vi "MainPanel.vi"() -> ()   [LabVIEW 2024]
panel:
  in  "Diagnose_Panel":enum32{"MAIN_PANEL", "COM_HANDLER"}(tab)
  in  "error name (type empty to clear)":string
  in  "Remove error":bool
  out "cem_off":bool
  out "cem_on":bool
  in  "UPDATE":bool
  in  "IGN_EN\nOn/Off":bool
  out "1_IGN":bool
  out "0_OFF":bool
  in  "GEAR SFT":i8(slide) scale=-1.0..6.0
  in  "PEDAL":i8(slide) scale=0.0..100.0
  out "power/torque/speed- graph":cluster{"power":i32, "torque":i32, "speed":u64}(graph)
  out "off":bool=TRUE
  out "on":bool
  in  "Send key check resp (auth req on(br.red)/off)":bool
  out "Security access status":string="N/A"
  out "?":string="    OCTAVIA III DIAGNOSE SERVICE"
  in  "STOP DIAG_SERVICE":bool
  in  "milliseconds to wait":u32=200
  out "key":u64
  out "seed":u64
  in  "GET security acces data":bool
  in  "Cluster":T1
  out "stop":bool=TRUE
  out "run":bool
  out "engine_info.speed":u64(knob) caption="km/h" scale=0.0..260.0 scale format="%#_3g"
  out "engine_info.rpm":u64(knob) caption="rpm" scale=0.0..6000.0 scale format="%#_5g"
  out "engine_info.coolant_temp":i32(slide) caption="°C" scale=50.0..130.0
  in  "Start/Stop measurement":bool
  out "engine_info.fuel_consumtion":dbl(slide) caption="l/100km" scale=0.0..30.0
  out "power_supply":dbl(knob) caption="V" scale=0.0..18.0
  out "ign_stat":string
  out "torque (Nm)":i32
  out "power (hp)":i32
  out "rpm":u64
  out "speed (km/h)":u64
  out "pedal_lvl (%)":i32
  out "GEAR":string
  out "fuel_consumtion (l/100km)":dbl
  out "oil_level (%)":i32
  out "coolant_level (%)":i32
  out "coolant_temp (°C)":i32
  out "voltage (V)":dbl
  in  "Set_Ped_EN":bool
  in  "Chng_Gear_EN":bool
  in  "IGNITION\nOFF_0/IGN_1":bool
  out "error_memory":string
  out "error_log":string
  out "error_input":string
  in  "update_err_mem":bool
  in  "update_err_input":bool
  in  "update_err_log":bool
  in  "CLR ERR MEM":bool
  in  "CLR ERR LOG":bool
  in  "CLR ERR INPUT":bool
  out "ceg_on":bool
  out "ceg_off":bool
  out "cei_on":bool
  out "cei_off":bool
  in  "oil_level":i32
  in  "cool_lvl":i32
  in  "voltage":i32
  in  "set cool lvl":bool
  in  "set voltage":bool
  in  "set oil lvl":bool
  in  "Array":cluster{"String":string, "Boolean":bool}[](array[cluster])=[{"String"="EngErr_RpmSensorMalfunction", "Boolean"=FALSE}, {"String"="EngErr_FuelConsmUnav", "Boolean"=FALSE}, {"String"="EngErr_SpdmtrFault\n                0xE0112:  \"EngErr_SpdmtrFault\",\n", "Boolean"=FALSE}, {"String"="EngErr_EngCoolOverheat", "Boolean"=FALSE}, {"String"="EngErr_OilLvlLow", "Boolean"=FALSE}, {"String"="EngErr_CoolLvlLow", "Boolean"=FALSE}, {"String"="EngErr_IgnMalfunction", "Boolean"=FALSE}, {"String"="EngErr_Malfunction_Injector_1", "Boolean"=FALSE}, {"String"="EngErr_Malfunction_Injector_2", "Boolean"=FALSE}, {"String"="EngErr_Malfunction_Injector_3", "Boolean"=FALSE}, {"String"="EngErr_Malfunction_Injector_4", "Boolean"=FALSE}, {"String"="ComErr_CanErr_LossOfComm", "Boolean"=FALSE}, {"String"="ComErr_CanErr_Overvoltage", "Boolean"=FALSE}, {"String"="ComErr_CanErr_Undervoltage", "Boolean"=FALSE}, {"String"="ElErr_Overvoltage", "Boolean"=FALSE}, {"String"="ElErr_Undervoltage", "Boolean"=FALSE}]
  in  "Inject errors":bool
  out "Injected":bool
  out "no.of.errs":i32
  out "update_error_memory":bool
  out "update_error_log":bool
  out "update_error_input":bool
  out "put_ign_stat_header":string="N/A"
  out "get_ignition_status_header":string
  out "get_sec_stat_header":string="N/A"
  in  "API_KEY":string="cheia04042025tema2restfulapi"
  out "get_key_headers":string="N/A"
  out "put_send_key_header":string="N/A"
  out "get_engine_info_header":string
  out "get_power_supply_header":string
  out "put_gear_change_header":string="N/A"
  out "put_pedal_lvl_header":string="N/A"
  out "get_error_memory_header":string
  out "get_error_log_header":string
  out "get_error_input_header":string
  out "delete_error_memory_header":string="N/A"
  out "delete_error_log_header":string="N/A"
  out "delete_error_inj_header":string="N/A"
  out "put_manipulate_oil_lvl_header":string="N/A"
  out "put_manipulate_voltage_header":string="N/A"
  out "put_manipulate_coolant_lvl_header":string="N/A"
  out "post_error_input_header":string="N/A"
  out "delete_clear_specific_error_header":string="N/A"
  # "Error manager"
  # "COCKPIT"
  # "-UPDATE/DELETE-"
  # "enabled/disabled"
  # "Security access"
  # "-UPDATE/DELETE-"
  # "enabled/disabled"
  # "-UPDATE/DELETE-"
  # "enabled/disabled"
  # "Delete specific error"
  # "CONTROLS (PUT)"
  # "Params"
  # "Manipulate values"
  # "to set errors"
  # "oil: 0-150 %\ncool: 0-150 %\nvoltage: 0-20 V"
  # "Error Injection(POST)"
  # "Click red circle\nto enable/disable\nauthentification\nrequest."
  # "GET REQUESTS"
  # "PUT REQUESTS"
  # "DELETE REQUESTS"
  # "DELETE REQUESTS"
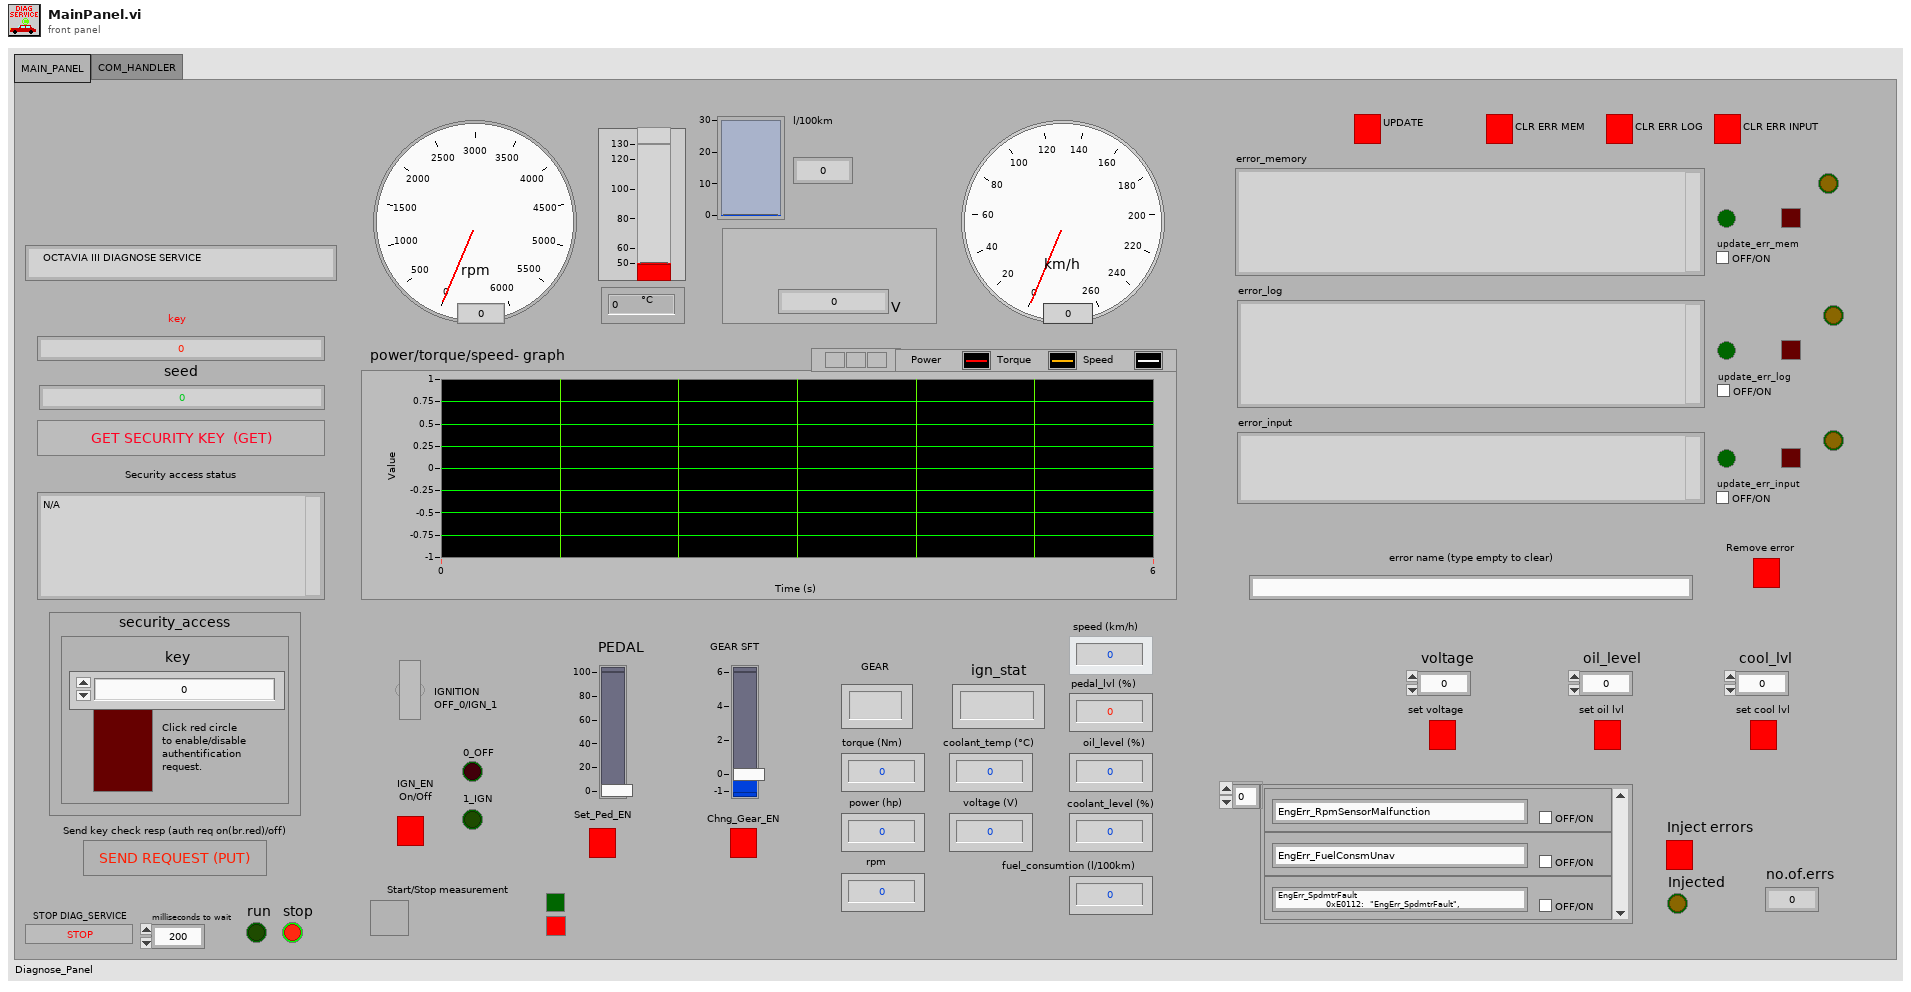
[diagram p1: front panel]
types:
  T1 = cluster{"security_access":cluster{"auth_request":bool, "key":u64}}
  T2 = cluster{"engine_info":cluster{"rpm":u64, "speed":u64, "gear":string, "power":i32, "torque":i32, "fuel_consumtion":dbl, "coolant_temp":i32, "coolant_level":i32, "oil_level":i32, "pedal_lvl":i32}}
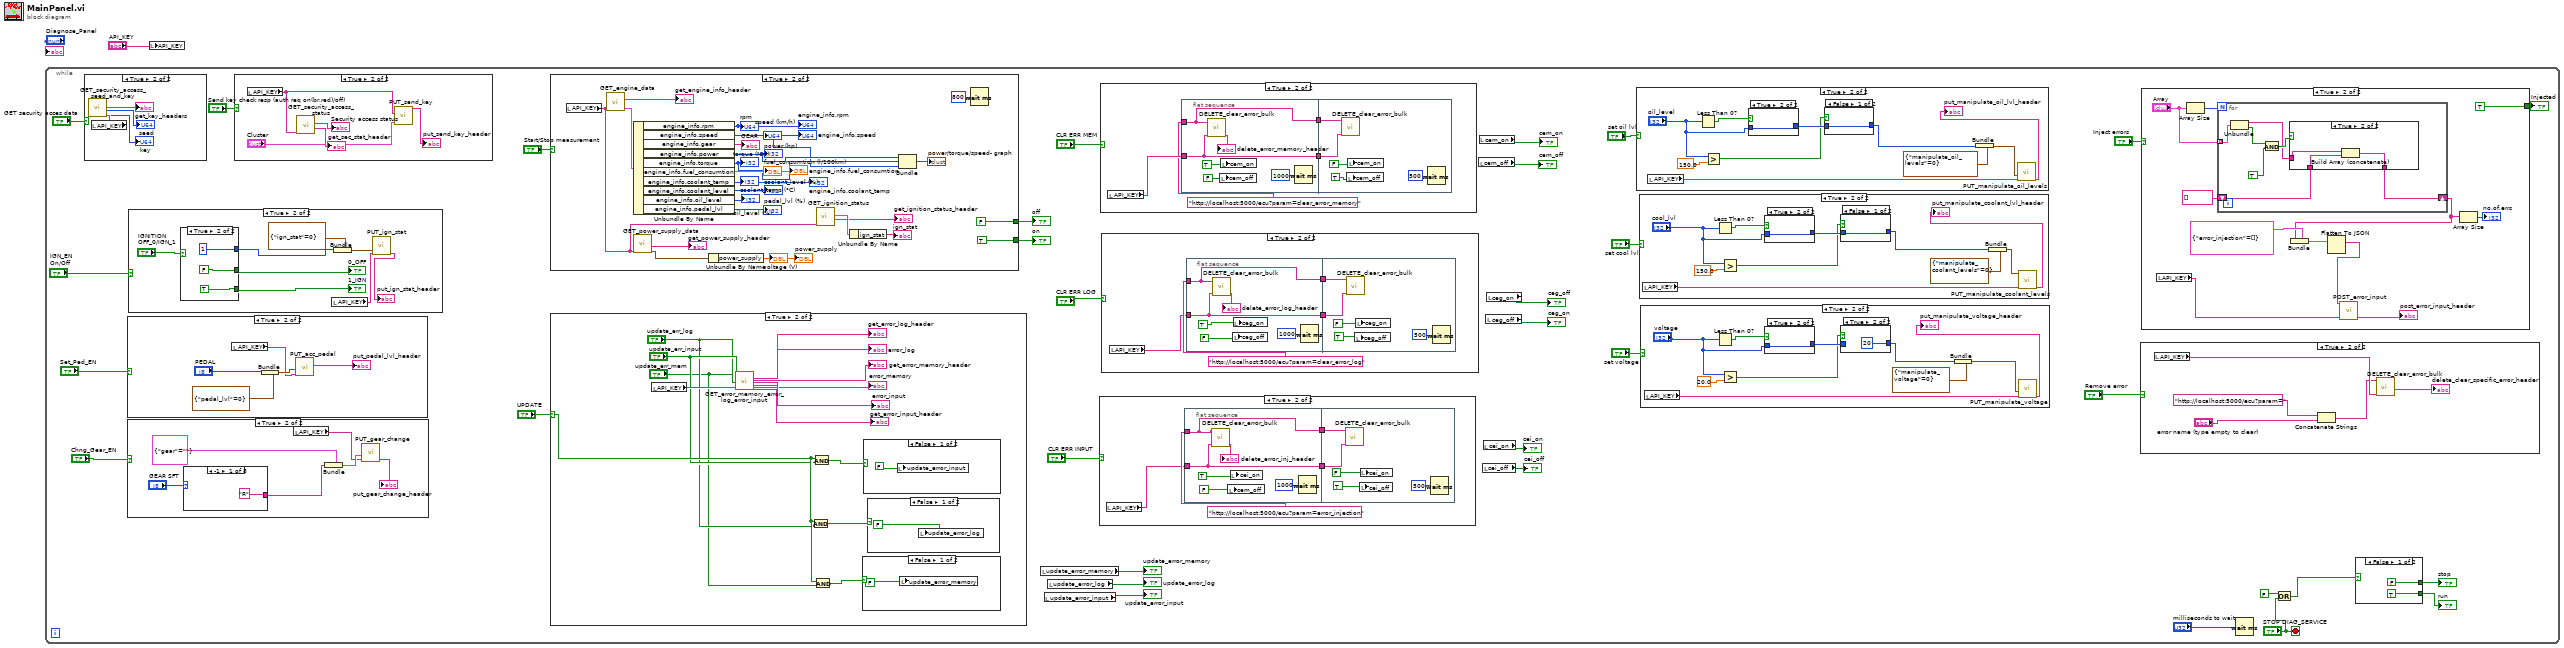
[diagram p0: block diagram]
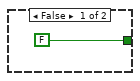
[diagram p3: hidden frame]
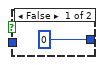
[diagram p7: hidden frame]
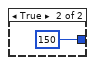
[diagram p9: hidden frame]
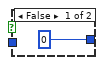
[diagram p10: hidden frame]
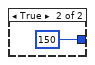
[diagram p12: hidden frame]
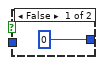
[diagram p13: hidden frame]
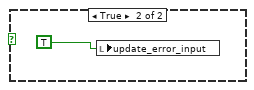
[diagram p18: hidden frame]
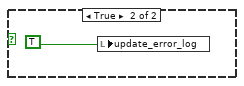
[diagram p19: hidden frame]
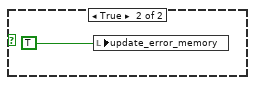
[diagram p20: hidden frame]
diagram:
  n1 = while {
    stop <- "STOP DIAG_SERVICE" stop-if-true
    n2 = case shown="True" "GET security acces data" {
      frame False {
      }
      frame True {
        n3 = local read "API_KEY"() -> (w240:string)
        n4 = call "GET_security_access_seed_and_key.vi"("API Key"=w240) -> ("key"=→"key":u64, "seed"=→"seed":u64, "headers"=→"get_key_headers":string)  [unwired: 5 in, 3 out]
      }
    }
    n5 = case shown="True" "Set_Ped_EN" {
      frame False {
      }
      frame True {
        n6 = local read "API_KEY"() -> (w184:string)
        n7 = Bundle(cluster=cluster{"pedal_lvl":i8} {"pedal_lvl"=0}, "pedal_lvl"="PEDAL") -> (w187:cluster{"pedal_lvl":i8})
        n8 = call "PUT_acc_pedal.vi"("API Key"=w184, "Cluster"=w187) -> ("headers"=→"put_pedal_lvl_header":string)  [unwired: 7 in, 2 out]
      }
    }
    n9 = case shown="True" "Chng_Gear_EN" {
      frame False {
      }
      frame True {
        n10 = case shown="-1" "GEAR SFT" {
          tunnel: ["R" "N" "1" "2" "3" "4" "5" "6"] -> w174
          frame -1 {
          }
          frame 0, Default {
          }
          frame 1 {
          }
          frame 2 {
          }
          frame 3 {
          }
          frame 4 {
          }
          frame 5 {
          }
          frame 6 {
          }
        }
        n11 = local read "API_KEY"() -> (w170:string)
        n12 = Bundle(cluster=cluster{"gear":string} {"gear"=""}, "gear"=w174) -> (w173:cluster{"gear":string})
        n13 = call "PUT_gear_change.vi"("API Key"=w170, "Cluster"=w173) -> ("headers"=→"put_gear_change_header":string)  [unwired: 7 in, 2 out]
      }
    }
    n14 = case shown="True" "IGN_EN\nOn/Off" {
      frame False {
      }
      frame True {
        n15 = case shown="True" "IGNITION\nOFF_0/IGN_1" {
          tunnel: [0 1] -> w192
          tunnel: [TRUE FALSE] -> w191
          tunnel: [FALSE TRUE] -> w195
          frame False {
          }
          frame True {
          }
        }
        "0_OFF" <- w191
        "1_IGN" <- w195
        n16 = local read "API_KEY"() -> (w190:string)
        n17 = Bundle(cluster=cluster{"ign_stat":i32} {"ign_stat"=0}, "ign_stat"=w192) -> (w193:cluster{"ign_stat":i32})
        n18 = call "PUT_ign_stat.vi"("API Key"=w190, "Cluster"=w193) -> ("headers"=→"put_ign_stat_header":string)  [unwired: 7 in, 2 out]
      }
    }
    n19 = case shown="True" "Send key check resp (auth req on(br.red)/off)" {
      frame False {
      }
      frame True {
        n20 = local read "API_KEY"() -> (w232:string)
        n21 = call "GET_security_access_status.vi"("API Key"=w232) -> ("headers"=→"get_sec_stat_header":string, "body"=→"Security access status":string)  [unwired: 8 in, 1 out]
        n22 = call "PUT_send_key.vi"("Cluster"="Cluster", "API Key"=w232) -> ("headers"=→"put_send_key_header":string)  [unwired: 8 in, 1 out]
      }
    }
    n23 = case shown="True" "Start/Stop measurement" {
      tunnel: [TRUE FALSE] -> w25
      tunnel: [FALSE TRUE] -> w24
      frame False {
      }
      frame True {
        n24 = local read "API_KEY"() -> (w209:string)
        n25 = call "GET_engine_data.vi"("API Key"=w209) -> ("engine info"=w226:T2, "headers"=→"get_engine_info_header":string)  [unwired: 8 in, 1 out]
        n26 = call "GET_power_supply_data.vi"("API Key"=w209) -> ("power_suppy"=w216:cluster{"power_supply":dbl}, "headers"=→"get_power_supply_header":string)  [unwired: 8 in, 1 out]
        n27 = Unbundle By Name(w226) -> ("engine_info.rpm"=→"rpm" →"engine_info.rpm":u64, "engine_info.speed"=w212:u64, "engine_info.gear"=→"GEAR":string, "engine_info.power"=w214:i32, "engine_info.torque"=w213:i32, "engine_info.fuel_consumtion"=→"fuel_consumtion (l/100km)" →"engine_info.fuel_consumtion":dbl, "engine_info.coolant_temp"=→"coolant_temp (°C)" →"engine_info.coolant_temp":i32, "engine_info.coolant_level"=→"coolant_level (%)":i32, "engine_info.oil_level"=→"oil_level (%)":i32, "engine_info.pedal_lvl"=→"pedal_lvl (%)":i32)
        "speed (km/h)" <- w212
        "power (hp)" <- w214
        "torque (Nm)" <- w213
        "engine_info.speed" <- w212
        n28 = Unbundle By Name(w216) -> ("power_supply"=→"voltage (V)" →"power_supply":dbl)
        n29 = call "GET_ignition_status.vi"("API Key"=w209) -> ("headers"=→"get_ignition_status_header":string, "ign_stat"=w208:cluster{"ign_stat":string})  [unwired: 8 in, 1 out]
        n30 = Unbundle By Name(w208) -> ("ign_stat"=→"ign_stat":string)
        n31 = Bundle("power"=w214, "torque"=w213, "speed"=w212) -> (→"power/torque/speed- graph":cluster{"power":i32, "torque":i32, "speed":u64})  [unwired: 1 in]
        n32 = Wait (ms)(milliseconds to wait=u32 800) -> ()  [unwired: 1 out]
      }
    }
    "on" <- w24
    "off" <- w25
    n33 = case shown="True" "UPDATE" {
      selector: "UPDATE" -> [_ w156]
      frame False {
      }
      frame True {
        n34 = local read "API_KEY"() -> (w157:string)
        n35 = call "GET_error_memory_error_log_error_input.vi"("update_err_log"="update_err_log", "update_err_input"="update_err_input", "update_err_mem"="update_err_mem", "API Key"=w157) -> ("body_error_log"=→"error_log":string, "get_error_memory"=→"get_error_memory_header":string, "body_error_input"=→"error_input":string, "get_error_log_header"=→"get_error_log_header":string, "body_error_memory"=→"error_memory":string, "get_error_input_header"=→"get_error_input_header":string)  [unwired: 18 in]
        n36 = And(x=w156, y="update_err_log") -> (x .and. y?=w154:bool)
        n37 = And(x=w156, y="update_err_input") -> (x .and. y?=w155:bool)
        n38 = And(x=w156, y="update_err_mem") -> (x .and. y?=w153:bool)
        n39 = case shown="False" w153 {
          frame False {
            n40 = local write "update_error_memory"(FALSE) -> ()
          }
          frame True {
            n41 = local write "update_error_memory"(TRUE) -> ()
          }
        }
        n42 = case shown="False" w155 {
          frame False {
            n43 = local write "update_error_input"(FALSE) -> ()
          }
          frame True {
            n44 = local write "update_error_input"(TRUE) -> ()
          }
        }
        n45 = case shown="False" w154 {
          frame False {
            n46 = local write "update_error_log"(FALSE) -> ()
          }
          frame True {
            n47 = local write "update_error_log"(TRUE) -> ()
          }
        }
      }
    }
    n48 = local read "update_error_memory"() -> (→"update_error_memory":bool)
    n49 = local read "update_error_input"() -> (→"update_error_input":bool)
    n50 = local read "update_error_log"() -> (→"update_error_log":bool)
    n51 = case shown="True" "CLR ERR INPUT" {
      frame False {
      }
      frame True {
        n52 = local read "API_KEY"() -> (w105:string)
        n53 = flat-sequence {
          tunnel: w105 -> [w114]
          tunnel: [w114] -> w108
          tunnel: "http://localhost:5000/ecu?param=error_injection" ("url") -> [w111]
          tunnel: [w111] -> w107
          tunnel: w108 -> [w119]
          tunnel: w107 -> [w117]
          frame #0 {
            n54 = call "DELETE_clear_error_bulk.vi"("API Key"=w114, "url"=w111) -> ("delete_error_"=→"delete_error_inj_header":string)  [unwired: 8 in, 1 out]
            n55 = local write "cem_off"(FALSE) -> ()
            n56 = local write "cei_on"(TRUE) -> ()
            n57 = Wait (ms)(milliseconds to wait=u32 1000) -> ()  [unwired: 1 out]
          }
          frame #1 {
            n58 = call "DELETE_clear_error_bulk.vi"("API Key"=w119, "url"=w117) -> ()  [unwired: 8 in, 2 out]
            n59 = local write "cei_off"(TRUE) -> ()
            n60 = local write "cei_on"(FALSE) -> ()
            n61 = Wait (ms)(milliseconds to wait=u32 500) -> ()  [unwired: 1 out]
          }
        }
      }
    }
    n62 = case shown="True" "CLR ERR MEM" {
      frame False {
      }
      frame True {
        n63 = local read "API_KEY"() -> (w138:string)
        n64 = flat-sequence {
          tunnel: w138 -> [w144]
          tunnel: [w144] -> w137
          tunnel: "http://localhost:5000/ecu?param=clear_error_memory" ("url") -> [w141]
          tunnel: [w141] -> w135
          tunnel: w137 -> [w149]
          tunnel: w135 -> [w147]
          frame #0 {
            n65 = call "DELETE_clear_error_bulk.vi"("API Key"=w144, "url"=w141) -> ("delete_error_"=→"delete_error_memory_header":string)  [unwired: 8 in, 1 out]
            n66 = local write "cem_off"(FALSE) -> ()
            n67 = local write "cem_on"(TRUE) -> ()
            n68 = Wait (ms)(milliseconds to wait=u32 1000) -> ()  [unwired: 1 out]
          }
          frame #1 {
            n69 = call "DELETE_clear_error_bulk.vi"("API Key"=w149, "url"=w147) -> ()  [unwired: 8 in, 2 out]
            n70 = local write "cem_off"(TRUE) -> ()
            n71 = local write "cem_on"(FALSE) -> ()
            n72 = Wait (ms)(milliseconds to wait=u32 500) -> ()  [unwired: 1 out]
          }
        }
      }
    }
    n73 = case shown="True" "CLR ERR LOG" {
      frame False {
      }
      frame True {
        n74 = local read "API_KEY"() -> (w120:string)
        n75 = flat-sequence {
          tunnel: w120 -> [w129]
          tunnel: [w129] -> w123
          tunnel: "http://localhost:5000/ecu?param=clear_error_log" ("url") -> [w126]
          tunnel: [w126] -> w122
          tunnel: w123 -> [w134]
          tunnel: w122 -> [w132]
          frame #0 {
            n76 = call "DELETE_clear_error_bulk.vi"("API Key"=w129, "url"=w126) -> ("delete_error_"=→"delete_error_log_header":string)  [unwired: 8 in, 1 out]
            n77 = local write "ceg_off"(FALSE) -> ()
            n78 = local write "ceg_on"(TRUE) -> ()
            n79 = Wait (ms)(milliseconds to wait=u32 1000) -> ()  [unwired: 1 out]
          }
          frame #1 {
            n80 = call "DELETE_clear_error_bulk.vi"("API Key"=w134, "url"=w132) -> ()  [unwired: 8 in, 2 out]
            n81 = local write "ceg_off"(TRUE) -> ()
            n82 = local write "ceg_on"(FALSE) -> ()
            n83 = Wait (ms)(milliseconds to wait=u32 500) -> ()  [unwired: 1 out]
          }
        }
      }
    }
    n84 = local read "cem_off"() -> (→"cem_off":bool)
    n85 = local read "cem_on"() -> (→"cem_on":bool)
    n86 = local read "cei_off"() -> (→"cei_off":bool)
    n87 = local read "cei_on"() -> (→"cei_on":bool)
    n88 = local read "ceg_off"() -> (→"ceg_on":bool)
    n89 = local read "ceg_on"() -> (→"ceg_off":bool)
    n90 = case shown="True" "set oil lvl" {
      frame False {
      }
      frame True {
        n91 = local read "API_KEY"() -> (w100:string)
        n92 = Less Than 0?(x="oil_level") -> (x < 0?=w96:bool)
        n93 = Greater?(x="oil_level", y=150.0) -> (0:w91:bool)
        n94 = case shown="True" w96 {
          tunnel: [0 w104] -> w93
          tunnel: "oil_level" -> [_ w104]
          frame False {
          }
          frame True {
          }
        }
        n95 = case shown="False" w91 {
          tunnel: [w101 150] -> w94
          tunnel: w93 -> [w101 _]
          frame False {
          }
          frame True {
          }
        }
        n96 = Bundle(cluster=cluster{"manipulate_oil_levels":i32} {"manipulate_oil_levels"=0}, "manipulate_oil_levels"=w94) -> (w97:cluster{"manipulate_oil_levels":i32})
        n97 = call "PUT_manipulate_oil_levels.vi"("API Key"=w100, "Cluster"=w97) -> ("headers"=→"put_manipulate_oil_lvl_header":string)  [unwired: 7 in, 2 out]
      }
    }
    n98 = case shown="True" "set cool lvl" {
      frame False {
      }
      frame True {
        n99 = local read "API_KEY"() -> (w86:string)
        n100 = Less Than 0?(x="cool_lvl") -> (x < 0?=w82:bool)
        n101 = Greater?(x="cool_lvl", y=150.0) -> (0:w79:bool)
        n102 = case shown="True" w82 {
          tunnel: [0 w90] -> w80
          tunnel: "cool_lvl" -> [_ w90]
          frame False {
          }
          frame True {
          }
        }
        n103 = case shown="False" w79 {
          tunnel: [w87 150] -> w78
          tunnel: w80 -> [w87 _]
          frame False {
          }
          frame True {
          }
        }
        n104 = Bundle(cluster=cluster{"manipulate_coolant_levels":i32} {"manipulate_coolant_levels"=0}, "manipulate_coolant_levels"=w78) -> (w83:cluster{"manipulate_coolant_levels":i32})
        n105 = call "PUT_manipulate_coolant_levels.vi"("API Key"=w86, "Cluster"=w83) -> ("headers"=→"put_manipulate_coolant_lvl_header":string)  [unwired: 8 in, 1 out]
      }
    }
    n106 = case shown="True" "set voltage" {
      frame False {
      }
      frame True {
        n107 = local read "API_KEY"() -> (w72:string)
        n108 = Less Than 0?(x="voltage") -> (x < 0?=w68:bool)
        n109 = Greater?(x="voltage", y=20.0) -> (0:w65:bool)
        n110 = case shown="True" w68 {
          tunnel: [0 w76] -> w66
          tunnel: "voltage" -> [_ w76]
          frame False {
          }
          frame True {
          }
        }
        n111 = case shown="True" w65 {
          tunnel: [w73 20] -> w63
          tunnel: w66 -> [w73 _]
          frame False {
          }
          frame True {
          }
        }
        n112 = Bundle(cluster=cluster{"manipulate_voltage":i32} {"manipulate_voltage"=0}, "manipulate_voltage"=w63) -> (w70:cluster{"manipulate_voltage":i32})
        n113 = call "PUT_manipulate_voltage.vi"("API Key"=w72, "Cluster"=w70) -> ("headers"=→"put_manipulate_voltage_header":string)  [unwired: 8 in, 1 out]
      }
    }
    n114 = case shown="True" "Remove error" {
      frame False {
      }
      frame True {
        n115 = local read "API_KEY"() -> (w39:string)
        n116 = Concatenate Strings("http://localhost:5000/ecu?param=" ("url"), "error name (type empty to clear)") -> (w36:string)
        n117 = call "DELETE_clear_error_bulk.vi"("API Key"=w39, "url"=w36) -> ("DELETE_clear_specific_error_header"=→"delete_clear_specific_error_header":string)  [unwired: 8 in, 1 out]
      }
    }
    n118 = case shown="True" "Inject errors" {
      tunnel: [FALSE TRUE] -> w6
      frame False {
      }
      frame True {
        n119 = local read "API_KEY"() -> (w43:string)
        n120 = Array Size(array="Array") -> (size(s)=w50:i32)
        n121 = for {
          N: w50 -> [_]
          tunnel: "Array" -> [w56] mode=indexing
          shift-right: [w53] -> w44
          shift-left: string[] [] -> [w52]
          n122 = Unbundle(w56) -> ("String"=w54:string, "Boolean"=w55:bool)
          n123 = And(x=w55, y=TRUE) -> (x .and. y?=w57:bool)
          n124 = case shown="True" w57 {
            tunnel: w54 -> [_ w62]
            tunnel: w52 -> [w59 w61]
            tunnel: [w59 w60] -> w53
            frame False {
            }
            frame True {
              n125 = Build Array (concatenate)(w62, w61) -> (w60:string[])
            }
          }
        }
        n126 = Bundle(cluster=cluster{"error_injection":string[]} {"error_injection"=[]}, "error_injection"=w44) -> (w46:cluster{"error_injection":string[]})
        n127 = Flatten To JSON(anything=w46) -> (JSON string=w42:string)  [unwired: 2 in, 1 out]
        n128 = call "POST_error_input.vi"("API Key"=w43, "JSON_input"=w42) -> ("headers"=→"post_error_input_header":string)  [unwired: 7 in, 2 out]
        n129 = Array Size(array=w44) -> (size(s)=→"no.of.errs":i32)
      }
    }
    "Injected" <- w6
    n130 = Wait (ms)(milliseconds to wait="milliseconds to wait") -> ()  [unwired: 1 out]
    n131 = Or(x=FALSE, y="STOP DIAG_SERVICE") -> (x .or. y?=w29:bool)
    n132 = case shown="False" w29 {
      tunnel: [FALSE TRUE] -> w28
      tunnel: [TRUE FALSE] -> w27
      frame False {
      }
      frame True {
      }
    }
    "stop" <- w28
    "run" <- w27
  }
  n133 = local write "API_KEY"("API_KEY") -> ()
